vi "Create Data (SubVI).vi"(11 "appended array":u8[][][](array[numeric])) -> (3 "appended array 2":u8[][][](array[numeric]))   [LabVIEW 2023]
uses:
  <vilib>/Analysis/baseanly.llb/Real Outer Product.vi
  <vilib>/Analysis/Matrix/Numeric/Conversions/Matrix To Array - RM.vi
  <vilib>/Analysis/NI_AALBase.lvlib
  <vilib>/Analysis/Matrix/NI_Matrix.lvlib
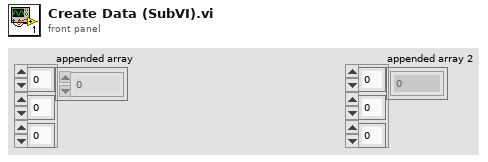
[diagram p1: front panel]
types:
  T1 = typedef "NI_Matrix.lvlib/RealMatrix.ctl" = dbl[][]
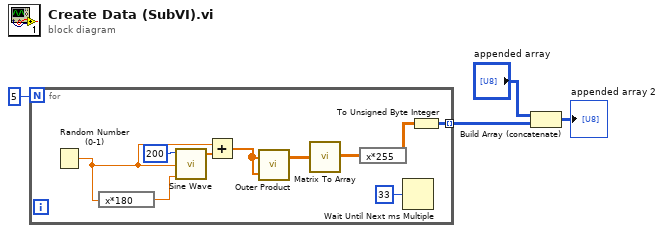
[diagram p0: block diagram]
diagram:
  n1 = for {
    N: 5 -> [_]
    tunnel: [w6] -> w3 mode=indexing
    n2 = Random Number (0-1)() -> (number: 0 to 1=w13:dbl)
    n3 = expression code="x*180"(w13) -> (w12:dbl)
    n4 = call <vilib>:"Sine Wave.vi"("samples"=200, "amplitude"=w13, "phase in"=w12) -> ("sine wave"=w14:dbl[])  [unwired: 2 in, 2 out]
    n5 = Add(x=w13, y=w14) -> (x+y=w11:dbl[])
    n6 = call-poly <vilib>:"Outer Product.vi"("Y Vector"=w11, "X Vector"=w11) -> ("Outer Product"=w10:T1)  [unwired: 1 out]
    n7 = call-poly <vilib>:"Matrix To Array.vi"("Real Matrix"=w10) -> ("Real 2D Array"=w7:dbl[][])
    n8 = expression code="x*255"(w7) -> (w5:dbl[][])
    n9 = Wait Until Next ms Multiple(millisecond multiple=u32 33) -> ()  [unwired: 1 out]
    n10 = To Unsigned Byte Integer(number=w5) -> (unsigned 8bit integer=w6:u8[][])
  }
  n11 = Build Array (concatenate)("appended array", w3) -> (→"appended array 2":u8[][][])
